vi "Configure Channel.vi"(8 "error in (no error)":errorcluster, 10 "DAQmx Task In":refnum<k21>, 11 "StrainChannel in":refnum<class "StrainChannel.lvclass">) -> (0 "error out":errorcluster, 2 "DAQmx Task":refnum<k21>)   [LabVIEW 2023, in "VolatusDAQConfig.lvlib" / "StrainChannel.lvclass"]
uses:
  StrainChannel.lvclass
  StrainChannel.lvclass/StrainChannel.ctl
  VolatusConfig/VolatusConfigElement/VolatusConfigElement.lvclass
  VolatusConfig/Channel/Channel Config.lvclass
  <vilib>/DAQmx/create/channels.llb/DAQmx Create Channel (AI-Strain-Strain Gage).vi
  C:/dev/volatus/mts-volatus-super/libs/lv-volatus/VolatusDAQConfig/DAQmxChannel/DAQmxChannel.lvclass
  C:/dev/volatus/mts-volatus-super/libs/lv-volatus/VolatusConfig/Channel/Channel Config.lvclass
  C:/dev/volatus/mts-volatus-super/libs/lv-volatus/VolatusConfig/VolatusConfigElement/VolatusConfigElement.lvclass
  C:/dev/volatus/mts-volatus-super/libs/lv-volatus/VolatusDAQConfig/StrainChannel/StrainChannel.lvclass
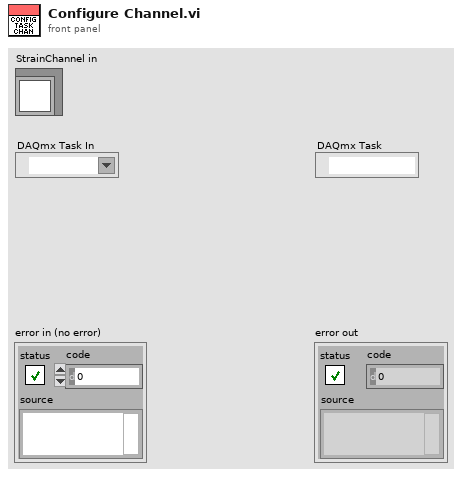
[diagram p1: front panel]
types:
  T1 = cluster{"strain configuration":i32, "lead wire resistance":dbl, "initial bridge voltage":dbl, "voltage excitation source":i32, "voltage excitation value":dbl}
  T2 = cluster{"gage factor":dbl, "nominal gage resistance":dbl, "poisson ratio":dbl}
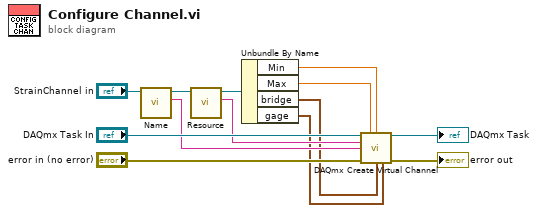
[diagram p0: block diagram]
diagram:
  n1 = call "Name.vi"("VolatusConfigElement in"="StrainChannel in") -> ("Name"=w7:string, "VolatusConfigElement out"=w9:refnum<class "StrainChannel.lvclass">)  [unwired: 8 in, 1 out]
  n2 = call "Resource.vi"("Channel in"=w9) -> ("Resource"=w6:string, "Channel out"=w5:refnum<class "StrainChannel.lvclass">)  [unwired: 8 in, 1 out]
  n3 = Unbundle By Name(w5) -> ("Min"=w1:dbl, "Max"=w2:dbl, "bridge"=w3:T1, "gage"=w4:T2)
  n4 = call-poly <vilib>:"DAQmx Create Virtual Channel.vi"("task in"="DAQmx Task In", "maximum value"=w2, "minimum value"=w1, "physical channels"=w6, "name to assign"=w7, "error in"="error in (no error)", "bridge information"=w3, "strain gage information"=w4) -> ("task out"=→"DAQmx Task":refnum<k21>, "error out"=→"error out":errorcluster)  [unwired: 6 in]
